vi "Cal String Parameter Adjust.vi"(5 "string in":string="Index=1\r\nchannelCalSourcing[01]=785\r\nchannelCalSourcing[02]=782\r\nchannelCalSourcing[03]=786\r\nchannelCalSourcing[04]=781\r\nchannelCalSourcing[05]=777\r\nchannelCalSourcing[06]=779\r\nchannelCalSourcing[07]=781\r\nchannelCalSourcing[08]=777\r\nchannelCalSourcing[09]=780\r\nchannelCalSourcing[10]=788\r\nchannelCalSourcing[11]=780\r\nchannelCalSourcing[12]=783\r\nchannelCalSourcing[13]=783\r\nchannelCalSourcing[14]=784\r\nchannelCalSourcing[15]=788\r\nchannelCalSourcing[16]=786\r\nchannelCalSourcing[17]=781\r\nchannelCalSourcing[18]=783\r\nchannelCalSourcing[19]=784\r\nchannelCalSourcing[20]=778\r\nchannelCalSourcing[21]=783\r\nchannelCalSourcing[22]=782\r\nchannelCalSourcing[23]=779\r\nchannelCalSourcing[24]=780\r\nchannelCalSourcing[25]=780\r\nchannelCalSourcing[26]=781\r\nchannelCalSinking[01]=810\r\nchannelCalSinking[02]=810\r\nchannelCalSinking[03]=812\r\nchannelCalSinking[04]=812\r\nchannelCalSinking[05]=803\r\nchannelCalSinking[06]=811\r\nchannelCalSinking[07]=806\r\nchannelCalSinking[08]=807\r\nchannelCalSinking[09]=813\r\nchannelCalSinking[10]=814\r\nchannelCalSinking[11]=810\r\nchannelCalSinking[12]=808\r\nchannelCalSinking[13]=810\r\nchannelCalSinking[14]=815\r\nchannelCalSinking[15]=816\r\nchannelCalSinking[16]=812\r\nchannelCalSinking[17]=809\r\nchannelCalSinking[18]=807\r\nchannelCalSinking[19]=811\r\nchannelCalSinking[20]=809\r\nchannelCalSinking[21]=816\r\nchannelCalSinking[22]=805\r\nchannelCalSinking[23]=811\r\nchannelCalSinking[24]=810\r\nchannelCalSinking[25]=816\r\nchannelCalSinking[26]=802") -> (2 "string out":string)   [LabVIEW 2010]
panel:
  in  "offset":i32
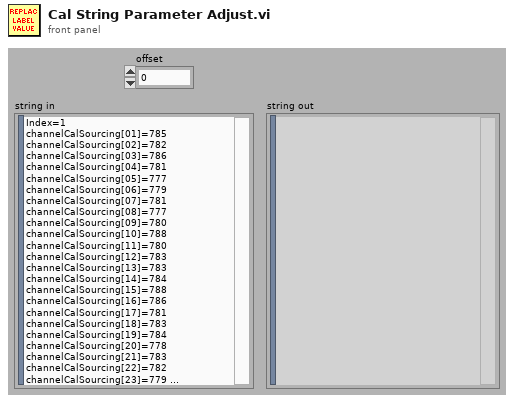
[diagram p1: front panel]
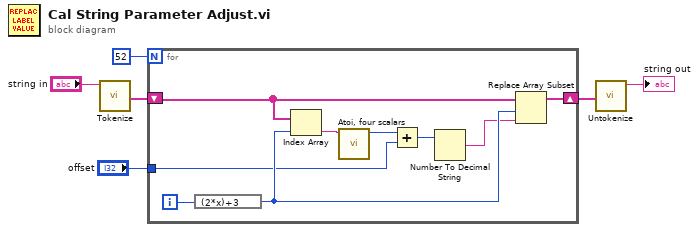
[diagram p0: block diagram]
diagram:
  n1 = call "Tokenize.vi"("input string"="string in") -> ("tokens"=w4:string[])  [unwired: 4 in, 2 out]
  n2 = for {
    N: 52 -> [_]
    shift-right: [w15] -> w3
    shift-left: w4 -> [w13]
    tunnel: "offset" -> [w7]
    i -> [w14]
    n3 = expression code="(2*x)+3"(w14) -> (w12:i32)
    n4 = Index Array(array=w13, index=w12) -> (element=w11:string)
    n5 = call "Atoi, four scalars.vi"("string 1"=w11) -> ("number 1"=w10:i32)  [unwired: 3 in, 3 out]
    n6 = Add(x=w10, y=w7) -> (x+y=w9:i32)
    n7 = Number To Decimal String(number=w9) -> (decimal integer string=w8:string)  [unwired: 1 in]
    n8 = Replace Array Subset(array=w13, new element=w8, index=w12) -> (w15:string[])
  }
  n9 = call "Untokenize.vi"("tokens"=w3) -> ("string out"=→"string out":string)  [unwired: 10 in]
